vi "PID Calculate.vi"(9 "dt (s)":dbl, 10 "Process Variable":dbl, 11 "PID Ref in":refnum<data-value>) -> (2 "output":dbl, 3 "PID Ref out":refnum<data-value>)   [LabVIEW 2019]
uses:
  Typedef/PID Controller State.ctl
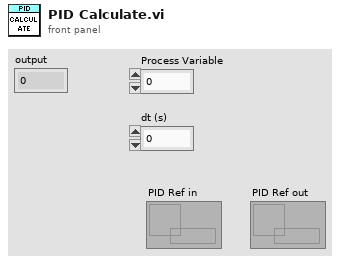
[diagram p1: front panel]
types:
  T1 = typedef "PID Controller State.ctl" = cluster{"PIDF Gains":cluster{"Kp":dbl, "Ki":dbl, "Kd":dbl, "Kf":dbl}, "Output Range":cluster{"output high":dbl, "output low":dbl}, "Profiled?":bool, "PID State":cluster{"iState":dbl, "dState":dbl, "Error [n-1]":dbl, "Output":dbl}, "Setpoint":dbl, "Profiled State":cluster{"Position":dbl, "Velocity":dbl}, "Profiled Contraints":cluster{"Max Velocity":dbl, "Max Acceleration":dbl}}
  T2 = cluster{"iState":dbl, "dState":dbl, "Error [n-1]":dbl, "Output":dbl}
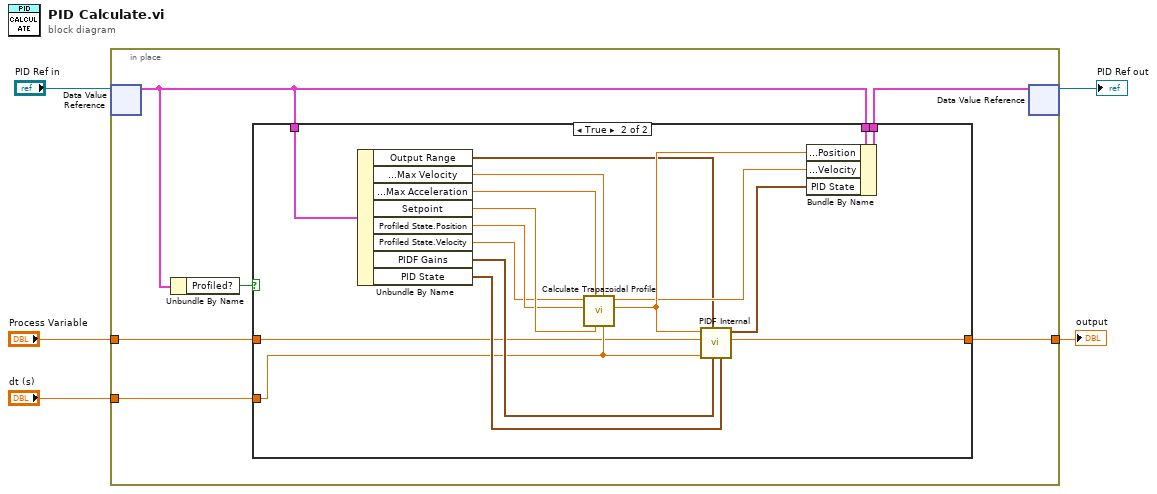
[diagram p0: block diagram]
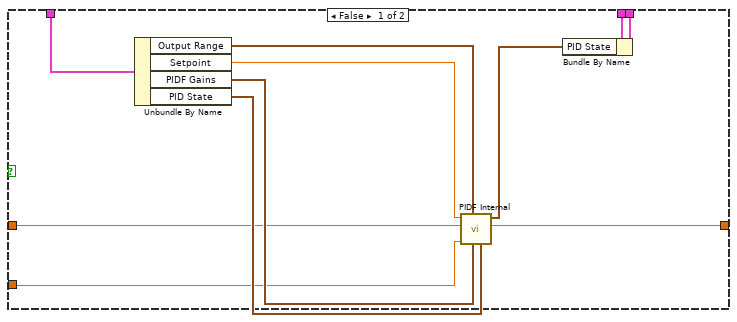
[diagram p2: hidden frame]
diagram:
  n1 = in-place {
    in-place-border: [w9] -> w3
    in-place-border: "dt (s)" -> [w8]
    in-place-border: "Process Variable" -> [w7]
    n2 = in-place-dvr #1("PID Ref in") -> (w6:T1)  [unwired: 1 out]
    n3 = Unbundle By Name(w6) -> ("Profiled?"=w10:bool)
    n4 = case shown="True" w10 {
      tunnel: w6 -> [w16 w28]
      tunnel: [w17 w27] -> w11
      tunnel: [w13 w26] -> w9
      tunnel: w8 -> [w14 w25]
      tunnel: w7 -> [w15 w24]
      tunnel: w6 -> [w12 w23]
      frame False {
        n5 = Unbundle By Name(w12) -> ("Output Range"=w22:cluster{"output high":dbl, "output low":dbl}, "Setpoint"=w20:dbl, "PIDF Gains"=w21:cluster{"Kp":dbl, "Ki":dbl, "Kd":dbl, "Kf":dbl}, "PID State"=w19:T2)
        n6 = call "PIDF Internal.vi"("PID State"=w19, "PIDF gains"=w21, "output range"=w22, "dt (s)"=w14, "process variable"=w15, "setpoint"=w20) -> ("output"=w13:dbl, "PID State"=w18:T2)  [unwired: 2 in, 2 out]
        n7 = Bundle By Name(cluster=w16, "PID State"=w18) -> (w17:T1)
      }
      frame True {
        n8 = Unbundle By Name(w23) -> ("Output Range"=w32:cluster{"output high":dbl, "output low":dbl}, "Profiled Contraints.Max Velocity"=w38:dbl, "Profiled Contraints.Max Acceleration"=w39:dbl, "Setpoint"=w37:dbl, "Profiled State.Position"=w36:dbl, "Profiled State.Velocity"=w35:dbl, "PIDF Gains"=w31:cluster{"Kp":dbl, "Ki":dbl, "Kd":dbl, "Kf":dbl}, "PID State"=w29:T2)
        n9 = call "Calculate Trapazoidal Profile.vi"("t"=w25, "Max Velocity"=w38, "Final Position"=w37, "Max Acceleration"=w39, "Initial Position"=w36, "Initial Velocity"=w35) -> ("Result Position"=w34:dbl, "Result Velocity"=w33:dbl)  [unwired: 4 in]
        n10 = call "PIDF Internal.vi"("PID State"=w29, "PIDF gains"=w31, "output range"=w32, "dt (s)"=w25, "process variable"=w24, "setpoint"=w34) -> ("output"=w26:dbl, "PID State"=w30:T2)  [unwired: 2 in, 2 out]
        n11 = Bundle By Name(cluster=w28, "Profiled State.Position"=w34, "Profiled State.Velocity"=w33, "PID State"=w30) -> (w27:T1)
      }
    }
    n12 = in-place-dvr #1(w11) -> (→"PID Ref out":refnum<data-value>)  [unwired: 1 out]
  }
  "output" <- w3
